vi "P29_Count1.vi"() -> ()   [LabVIEW 2022 SP3]
uses:
  <vilib>/MakerHub/LINX/Public/Peripherals/Digital/Digital Read 1 Chan.vi
  <vilib>/MakerHub/LINX/Public/Peripherals/Digital/Digital Write N Chans.vi
  <vilib>/MakerHub/LINX/Public/Peripherals/Digital/Digital Read N Chans.vi
  <vilib>/MakerHub/LINX/Private/Local IO/LinxDigitalWrite.vi
  <vilib>/MakerHub/LINX/Public/Utilities/Check Channel.vi
  <vilib>/MakerHub/LINX/Private/Local IO/LinxDigitalRead.vi
  <vilib>/MakerHub/LINX/Public/Utilities/Open Serial.vi
  <vilib>/MakerHub/LINX/Private/Utilties/Generate Error.vi
  <vilib>/MakerHub/LINX/LMH-LINX.lvlib
panel:
  out "a":bool
  out "g":bool
  out "d":bool
  out "b":bool
  out "c":bool
  out "f":bool
  out "e":bool
  in  "Serial Port":refnum<visa-resource-name>
  in  "Boolean 3":bool
  in  "RESET":bool
  in  "Boolean 2":bool
  in  "UP":bool
  in  "stop":bool
  out "Numeric":dbl
  in  "Boolean":bool
  in  "START / STOP":bool
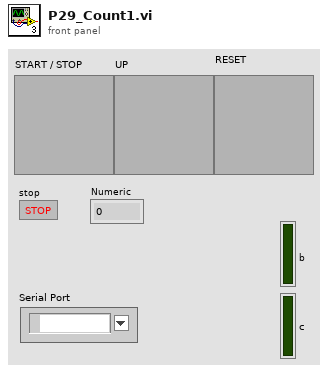
[diagram p1: front panel]
types:
  T1 = typedef "LMH-LINX.lvlib/LINX Ref.ctl" = cluster{"IO":T2, "Interface":T3, "LINX Device Config":T4}
  T2 = typedef "LMH-LINX.lvlib/Platform.ctl" = enum16{"Remote", "Local"}
  T3 = typedef "LMH-LINX.lvlib/Interface.ctl" = enum16{"Serial", "TCP"}
  T4 = typedef "LMH-LINX.lvlib/Device.lvlib/LINX Device Config.ctl" = cluster{"Interface":T3, "COM Port":refnum<visa-resource-name>, "TCP Configuration":T5, "Device Family":u8, "Device ID":u8, "Device Name":string, "TCP Ref":refnum<k5>, "Channels":T6}
  T5 = typedef "LMH-LINX.lvlib/Device.lvlib/TCP Config.ctl" = cluster{"IP Address":string, "Port":u16}
  T6 = typedef "LMH-LINX.lvlib/Channels.ctl" = cluster{"DI":u8[], "DO":u8[], "AI":u8[], "AO":u8[], "PWM":u8[], "QE":u8[], "UART":u8[], "I2C 2":u8[], "SPI":u8[], "CAN":u8[], "Servo":u8[], "AI Ref (V)":dbl, "AI Resolution (Bits)":u8, "AO Ref (V)":dbl, "AO Resolution (Bits)":u8}
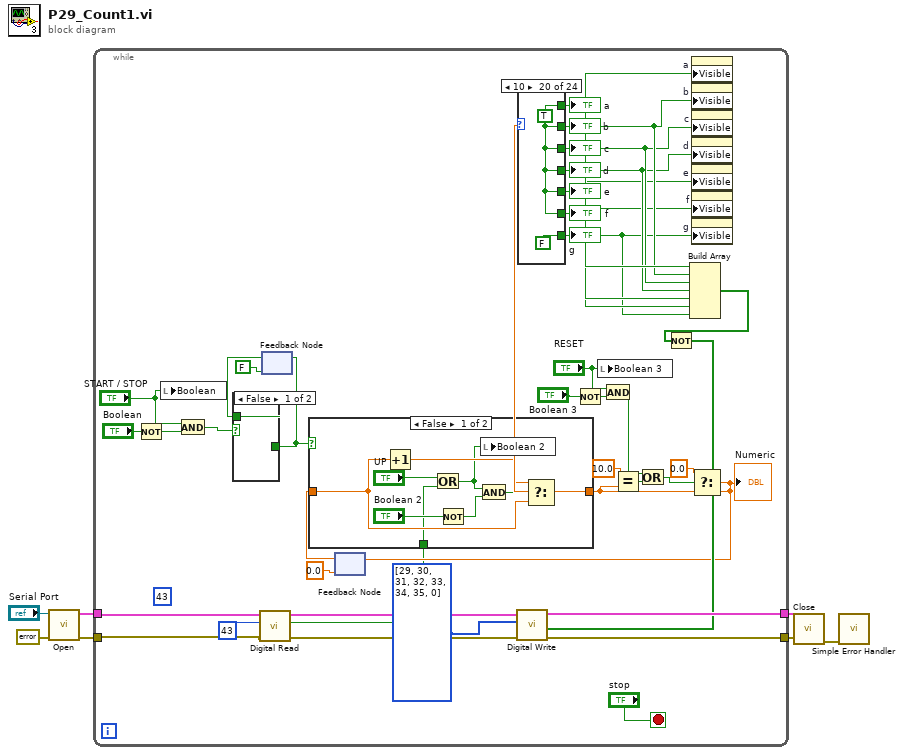
[diagram p0: block diagram]
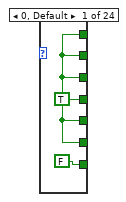
[diagram p2: hidden frame]
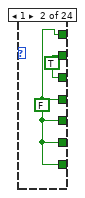
[diagram p3: hidden frame]
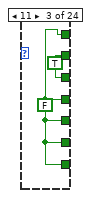
[diagram p4: hidden frame]
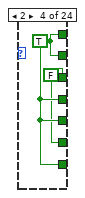
[diagram p5: hidden frame]
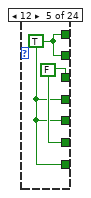
[diagram p6: hidden frame]
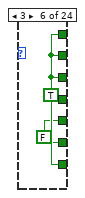
[diagram p7: hidden frame]
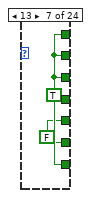
[diagram p8: hidden frame]
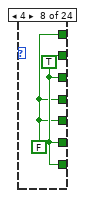
[diagram p9: hidden frame]
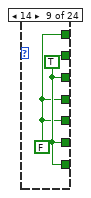
[diagram p10: hidden frame]
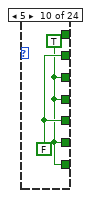
[diagram p11: hidden frame]
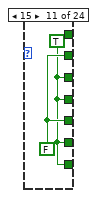
[diagram p12: hidden frame]
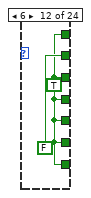
[diagram p13: hidden frame]
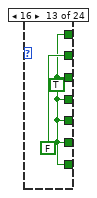
[diagram p14: hidden frame]
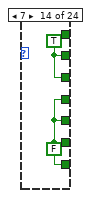
[diagram p15: hidden frame]
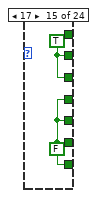
[diagram p16: hidden frame]
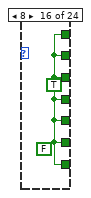
[diagram p17: hidden frame]
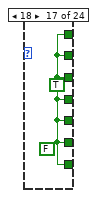
[diagram p18: hidden frame]
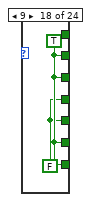
[diagram p19: hidden frame]
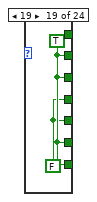
[diagram p20: hidden frame]
diagram:
  n1 = call-poly <vilib>:"Open.vi"("Error In"=errorcluster {"status"=FALSE, "code"=0, "source"=""}, "Serial Port"="Serial Port") -> ("Error Out"=w4:errorcluster, "LINX Resource"=w5:T1)  [unwired: 7 in, 1 out]
  n2 = while {
    tunnel: w5 -> [w24]
    tunnel: w4 -> [w23]
    tunnel: [w22] -> w2
    tunnel: [w21] -> w1
    stop <- "stop" stop-if-true
    (unwired) u8 43 ("DI Channel")
    n3 = Not(x="Boolean") -> (.not. x?=w45:bool)
    n4 = local write "Boolean"("START / STOP") -> ()
    n5 = And(x="START / STOP", y=w45) -> (x .and. y?=w39:bool)
    n6 = call-poly <vilib>:"Digital Read.vi"("Error In"=w23, "DI Channel"=u8 43, "LINX Resource"=w24) -> ("Error Out"=w26:errorcluster, "DI Value"=w15:bool, "LINX Resource"=w25:T1)  [unwired: 6 in]
    n7 = feedback #1(FALSE) -> (w38:bool)
    n8 = case shown="False" w39 {
      tunnel: [w92 w94] -> w37
      tunnel: w38 -> [w92 w93]
      frame False {
      }
      frame True {
        n9 = Not(x=w93) -> (.not. x?=w94:bool)
      }
    }
    n10 = feedback-in #1(w37) -> ()
    n11 = feedback #2(0.0) -> (w43:dbl)
    n12 = case shown="False" w37 {
      tunnel: [w101 w104] -> w33
      tunnel: w43 -> [w102 w105]
      tunnel: w15 -> [w95 _]
      frame False {
        n13 = Increment(x=w102) -> (x+1=w103:dbl)
        n14 = Or(x="UP", y=w95) -> (x .or. y?=w96:bool)
        n15 = Not(x="Boolean 2") -> (.not. x?=w99:bool)
        n16 = And(x=w96, y=w99) -> (x .and. y?=w98:bool)
        n17 = local write "Boolean 2"(w96) -> ()
        n18 = Select(t=w103, s=w98, f=w102) -> (s? t:f=w101:dbl)
      }
      frame True {
        n19 = Wait (ms)(milliseconds to wait=u32 500) -> ()  [unwired: 1 out]
        n20 = Increment(x=w105) -> (x+1=w104:dbl)
      }
    }
    n21 = Not(x="Boolean 3") -> (.not. x?=w28:bool)
    n22 = local write "Boolean 3"("RESET") -> ()
    n23 = And(x="RESET", y=w28) -> (x .and. y?=w27:bool)
    n24 = Equal?(x=10.0, y=w33) -> (x = y?=w32:bool)
    n25 = Or(x=w27, y=w32) -> (x .or. y?=w31:bool)
    n26 = Select(t=0.0, s=w31, f=w33) -> (s? t:f=w16:dbl)
    "Numeric" <- w16
    n27 = feedback-in #2(w16) -> ()
    n28 = case shown="10" w16 {
      tunnel: [w47 w48 w50 w53 w54 w57 w59 w60 w62 w64 w66 w68 w70 w73 w75 w76 w77 w79 w81 w83 w85 w86 w89 w91] -> w14
      tunnel: [w47 w48 w50 w52 w55 w56 w58 w61 w63 w64 w66 w68 w70 w72 w74 w76 w77 w79 w81 w83 w85 w86 w88 w90] -> w9
      tunnel: [w47 w49 w51 w53 w54 w57 w59 w61 w63 w65 w67 FALSE FALSE w73 w75 w76 w77 w79 w81 w83 w85 w87 w89 w91] -> w13
      tunnel: [w47 w49 w51 w52 w55 w57 w59 w61 w63 w64 w66 w68 w70 w73 w75 w76 w77 w79 w81 w83 w85 w87 w88 w91] -> w12
      tunnel: [w47 w48 w50 w53 w54 w57 w59 w60 w62 w64 w66 w68 w70 w72 w74 w76 w77 w78 w80 w83 w85 w86 w89 w91] -> w11
      tunnel: [w47 w48 w50 w53 w54 w56 w58 w60 w62 w65 w67 w68 w70 w72 w74 w76 w77 w78 w80 w83 w85 w86 w89 w90] -> w10
      tunnel: [FALSE w48 w50 w53 w54 w57 w59 w61 w63 w64 w66 w68 w70 w72 w74 w76 w77 w79 w81 FALSE FALSE w86 w89 w91] -> w8
      frame 0, Default {
        w47 = TRUE
      }
      frame 1 {
        w48 = FALSE
        w49 = TRUE
      }
      frame 11 {
        w50 = FALSE
        w51 = TRUE
      }
      frame 2 {
        w52 = FALSE
        w53 = TRUE
      }
      frame 12 {
        w55 = FALSE
        w54 = TRUE
      }
      frame 3 {
        w56 = FALSE
        w57 = TRUE
      }
      frame 13 {
        w58 = FALSE
        w59 = TRUE
      }
      frame 4 {
        w60 = FALSE
        w61 = TRUE
      }
      frame 14 {
        w62 = FALSE
        w63 = TRUE
      }
      frame 5 {
        w65 = FALSE
        w64 = TRUE
      }
      frame 15 {
        w67 = FALSE
        w66 = TRUE
      }
      frame 6 {
        w68 = TRUE
      }
      frame 16 {
        w70 = TRUE
      }
      frame 7 {
        w72 = FALSE
        w73 = TRUE
      }
      frame 17 {
        w74 = FALSE
        w75 = TRUE
      }
      frame 8 {
        (unwired) FALSE
        w76 = TRUE
      }
      frame 18 {
        (unwired) FALSE
        w77 = TRUE
      }
      frame 9 {
        w78 = FALSE
        w79 = TRUE
      }
      frame 19 {
        w80 = FALSE
        w81 = TRUE
      }
      frame 10 {
        w83 = TRUE
      }
      frame 20 {
        w85 = TRUE
      }
      frame 21 {
        w87 = TRUE
        w86 = FALSE
      }
      frame 22 {
        w88 = FALSE
        w89 = TRUE
      }
      frame 23 {
        w90 = FALSE
        w91 = TRUE
      }
    }
    "a" <- w14
    "g" <- w8
    "d" <- w11
    "b" <- w13
    "c" <- w12
    "f" <- w9
    "e" <- w10
    n29 = Build Array(w14, w13, w12, w11, w10, w9, w8) -> (w18:bool[])
    n30 = Not(x=w18) -> (.not. x?=w17:bool[])
    n31 = call-poly <vilib>:"Digital Write.vi"("Error In"=w26, "Values"=w17, "DO Channels"=u8[] [29, 30, 31, 32, 33, 34, 35, 0], "LINX Resource"=w25) -> ("Error Out"=w22:errorcluster, "LINX Resource"=w21:T1)  [unwired: 6 in]
    n32 = property on="a" class="Bool (strict)"("Visible"=w14) -> ()  [unwired: 2 in, 2 out]
    n33 = property on="b" class="Bool (strict)"("Visible"=w13) -> ()  [unwired: 2 in, 2 out]
    n34 = property on="c" class="Bool (strict)"("Visible"=w12) -> ()  [unwired: 2 in, 2 out]
    n35 = property on="d" class="Bool (strict)"("Visible"=w11) -> ()  [unwired: 2 in, 2 out]
    n36 = property on="e" class="Bool (strict)"("Visible"=w10) -> ()  [unwired: 2 in, 2 out]
    n37 = property on="f" class="Bool (strict)"("Visible"=w9) -> ()  [unwired: 2 in, 2 out]
    n38 = property on="g" class="Bool (strict)"("Visible"=w8) -> ()  [unwired: 2 in, 2 out]
  }
  n39 = call <vilib>:"Close.vi"("Error In"=w2, "LINX Resource"=w1) -> ("Error Out"=w3:errorcluster)  [unwired: 9 in]
  n40 = call <vilib>:"Simple Error Handler.vi"("error in (no error)"=w3) -> ()  [unwired: 4 in, 5 out]
